vi "FiberSpectrograph_issueCommand_captureSpectImage.vi"(8 "error in (no error)":errorcluster, 11 "command_captureSpectImage_Ctl":T1={"integrationTime"=0.0, "imageType"="                                                                                                                                                                                                                                                                ", "lamp"=""}) -> (0 "error out":errorcluster, 2 "function return":i32, 3 "command_captureSpectImage_Ctl out":T1={"integrationTime"=0.0, "imageType"="                                                                                                                                                                                                                                                                ", "lamp"=""})   [LabVIEW 2016, in "SALLV_FiberSpectrograph.lvlib"]
doc: "int FiberSpectrograph_shm_issueCommand_captureSpectImageLV(FiberSpectrograph_command_captureSpectImageLV *command_captureSpectImage_Ctl );"
uses:
  SALLV_FiberSpectrograph.lvlib
  DataTypes/command_captureSpectImage.ctl
  SALLV_FiberSpectrograph.so
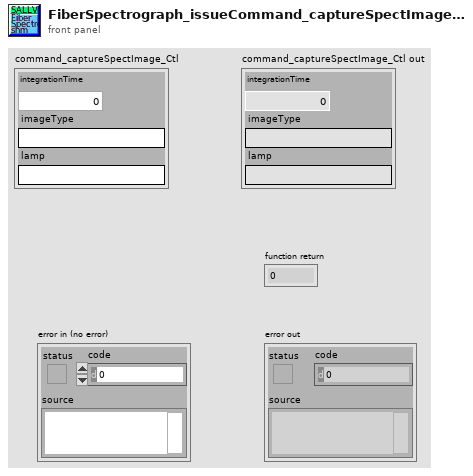
[diagram p1: front panel]
types:
  T1 = typedef "SALLV_FiberSpectrograph.lvlib/command_captureSpectImage.ctl" = cluster{"integrationTime":sgl, "imageType":string, "lamp":string}
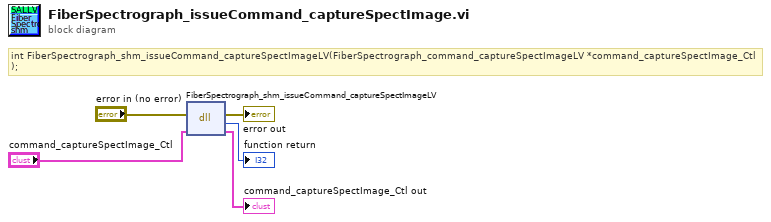
[diagram p0: block diagram]
diagram:
  # "int FiberSpectrograph_shm_issueCommand_captureSpectImageLV(FiberSpectrograph_command_captureSpectImageLV *command_captureSpectImage_Ctl );"
  n1 = dll-call lib="home/harini/SALLV_FiberSpectrograph/SALLV_FiberSpectrograph.*" fn="FiberSpectrograph_shm_issueCommand_captureSpectImageLV"(error in="error in (no error)", "command_captureSpectImage_Ctl"="command_captureSpectImage_Ctl") -> (error out=→"error out":errorcluster, →"function return":i32, "command_captureSpectImage_Ctl"=→"command_captureSpectImage_Ctl out":T1)  [unwired: 2 in, 1 out]
